vi "JSON to Schemes.vi"(11 "Material JSON":string) -> (0 "error out":errorcluster, 3 "Schemes":refnum<class "Material-Scheme.lvclass">[](array[class]))   [LabVIEW 2026, in "TSC Material Theme.lvlib" / "Material-Scheme.lvclass"]
doc: "Convert a JSON object to array of schemes.\n\n<b>Code Developed By:</b> +\nDaniel Coons +\nTechnology Service Corporation +\nwww.tsc.com/atcs"
uses:
  Material-Scheme.lvclass
  Serializer-Scheme/Serializer-Scheme.lvclass
  Serializer-Scheme/Serializer-Scheme.lvclass/Serializer-Scheme.ctl
  bcc1f051-5bb6-434e-b816-a57df783be2e.vi
  Serializer-Scheme/Set Name.vi
  <vilib>/JDP Science/JSONtext/Find Item.vi
  <vilib>/JDP Science/JSONtext/String Subset.vi
  <vilib>/JDP Science/JSONtext/Offset/Find Object Item Locations by Names.vi
  <vilib>/JDP Science/JSONtext/support/Quote and Escape JSON string.vi
  <vilib>/JDP Science/JSONtext/Next JSON Value.vi
  <vilib>/JDP Science/JSONtext/Parsing/Advance past whitespace.vi
  <vilib>/JDP Science/JSONtext/support/Commas Needed.vi
  <vilib>/JDP Science/JSONtext/Parsing/Advance past whitespace and comma.vi
  <vilib>/JDP Science/JSONtext/Parsing/Advance past next JSON Value (inlined COPY).vi
  <vilib>/JDP Science/JSONtext/Parsing/Advance past Item Name.vi
  <vilib>/JDP Science/JSONtext/support/quote and escape json string 2.vi
  <vilib>/JDP Science/JSONtext/Parsing/Advance past Line Ending.vi
  <vilib>/JDP Science/JSONtext/Parsing/Advance past String.vi
  <vilib>/JDP Science/JSONtext/Parsing/Advance past Number.vi
  <vilib>/JDP Science/JSONtext/Parsing/Parse Full Path or Item Name.vi
  <vilib>/JDP Science/JSONtext/Parsing/Advance past Array.vi
  <vilib>/JDP Science/JSONtext/Parsing/Advance past Object.vi
  <vilib>/JDP Science/JSONtext/support/Error Cluster From Code.vi
  <vilib>/JDP Science/JSONtext/Offset/Find Item Locations by Path.vi
  <vilib>/JDP Science/JSONtext/Parsing/Parsing Error.vi
  <vilib>/JDP Science/JSONtext/JSON text to Variant.vi
  <vilib>/JDP Science/JSONtext/JSONtext.lvlib
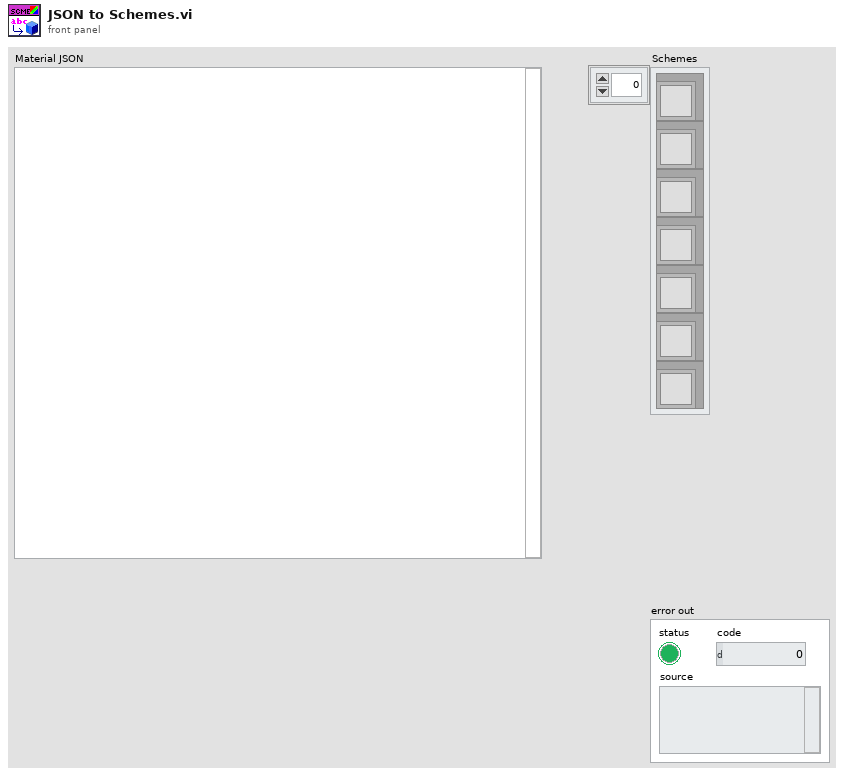
[diagram p1: front panel]
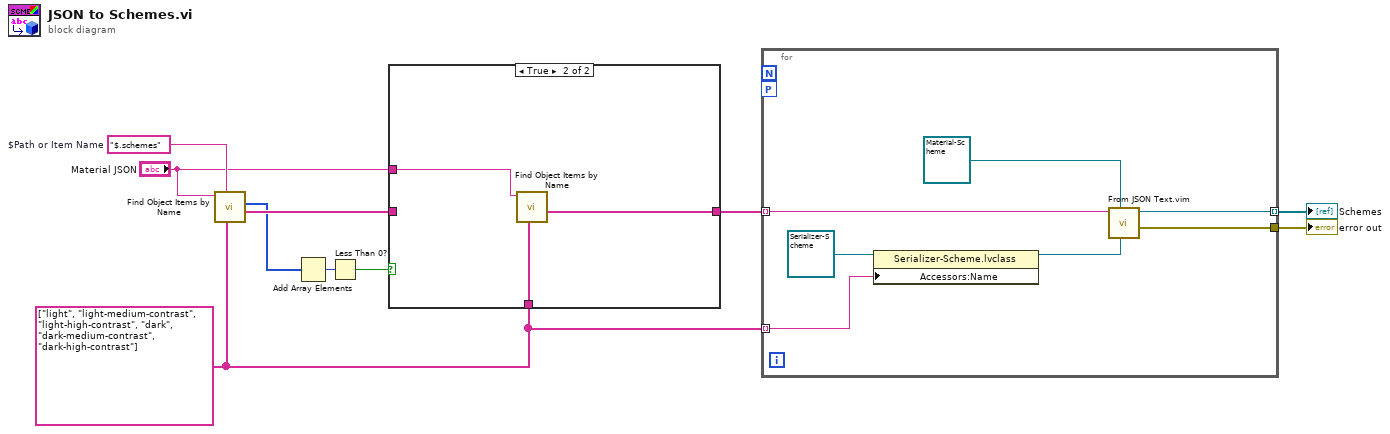
[diagram p0: block diagram]
diagram:
  w9 = "$.schemes"  # $Path or Item Name
  w5 = string[] ["light", "light-medium-contrast", "light-high-contrast", "dark", "dark-medium-contrast", "dark-high-contrast"] ("Item Names")
  n1 = call <vilib>:"Find Object Items by Name.vi"("Item Names"=w5, "$Path or Item Name"=w9, "JSON"="Material JSON") -> ("<JSON>"=w7:string[], "Offsets"=w3:i32[])  [unwired: 6 in, 1 out]
  n2 = Add Array Elements(numeric array=w3) -> (sum=w2:i32)
  n3 = Less Than 0?(x=w2) -> (x < 0?=w1:bool)
  n4 = case shown="True" w1 {
    tunnel: w7 -> [w11 _]
    tunnel: [w11 w12] -> w4
    tunnel: "Material JSON" -> [_ w14]
    tunnel: w5 -> [_ w13]
    frame False {
    }
    frame True {
      n5 = call <vilib>:"Find Object Items by Name.vi"("Item Names"=w13, "JSON"=w14) -> ("<JSON>"=w12:string[])  [unwired: 7 in, 2 out]
    }
  }
  n6 = for {
    tunnel: [w19] -> w8 mode=indexing
    tunnel: [w21] -> w10
    tunnel: w4 -> [w18] mode=indexing
    tunnel: w5 -> [w15] mode=indexing
    workers-P: _ -> [_]
    n7 = property class="Serializer-Scheme.lvclass"(reference=refnum<class "Serializer-Scheme.lvclass"> refnum ("TSC Material Theme.lvlib:Class 1.lvclass"), "Accessors:Name"=w15) -> (reference out=w16:refnum<class "Serializer-Scheme.lvclass">)  [unwired: 1 in, 1 out]
    n8 = call "From JSON Text.vim"("LVClass Serializer"=w16, "Data Type and Default Value"=refnum<class "Material-Scheme.lvclass"> refnum ("TSC Material Theme.lvlib:Material-Scheme"), "JSON"=w18) -> ("error out"=w21:errorcluster, "Data out"=w19:refnum<class "Material-Scheme.lvclass">)  [unwired: 7 in]
  }
  "Schemes" <- w8
  "error out" <- w10
